vi "KeywordWrite.vi"(0 "Crate":string, 2 "Keyword":string, 3 "Value":string, 7 "Service":string, 9 "error in (no error)":errorcluster) -> (1 "done?":refnum<k4>, 6 "error out":errorcluster)   [LabVIEW 2009]
uses:
  Controls/KeywordCommand.ctl
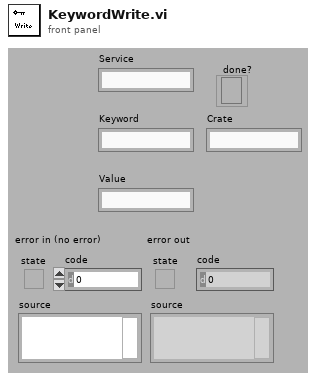
[diagram p1: front panel]
types:
  T1 = typedef "KeywordCommand.ctl" = cluster{"Command":enum16{"READ", "READBINARY", "WRITE", "QUIT"}, "Service":string, "Keyword":string, "Value":string, "done?":refnum<k4>}
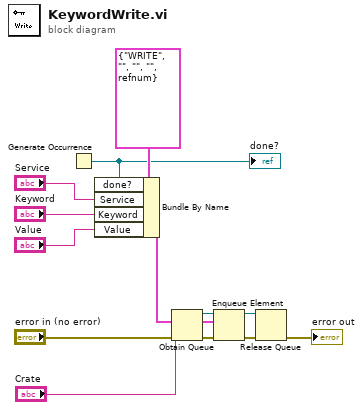
[diagram p0: block diagram]
diagram:
  n1 = Generate Occurrence() -> (w1:refnum<k4>)
  "done?" <- w1
  n2 = Bundle By Name(cluster=T1 {"Command"=enum."WRITE", "Service"="", "Keyword"="", "Value"="", "done?"=refnum} ("KeywordCommand"), "done?"=w1, "Service"="Service", "Keyword"="Keyword", "Value"="Value") -> (w6:T1)
  n3 = Obtain Queue(name (unnamed)="Crate", element data type=w6, error in (no error)="error in (no error)") -> (queue out=w7:refnum<queue>, error out=w8:errorcluster)  [unwired: 2 in, 1 out]
  n4 = Enqueue Element(queue=w7, element=w6, error in (no error)=w8) -> (queue out=w4:refnum<queue>, error out=w5:errorcluster)  [unwired: 2 out]
  n5 = Release Queue(queue=w4, error in (no error)=w5) -> (error out=→"error out":errorcluster)  [unwired: 3 out]
